vi "RotateX.vi"(8 "error in (no error)":errorcluster, 9 "radians":dbl, 10 "Modelview in":dbl[][](array[numeric])=[[1.0, 0.0, 0.0, 0.0], [0.0, 1.0, 0.0, 0.0], [0.0, 0.0, 1.0, 0.0], [0.0, 0.0, 0.0, 1.0]], 11 "3D Scene in":refnum<class "3D Scene.lvclass">) -> (0 "error out":errorcluster, 2 "Modelview out":dbl[][](array[numeric]), 3 "3D Scene out":refnum<class "3D Scene.lvclass">)   [LabVIEW 2015, in "3D Scene.lvclass"]
uses:
  3D Scene.lvclass
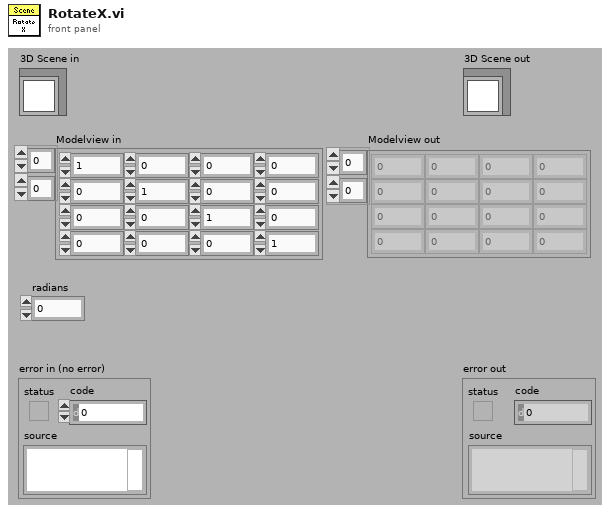
[diagram p1: front panel]
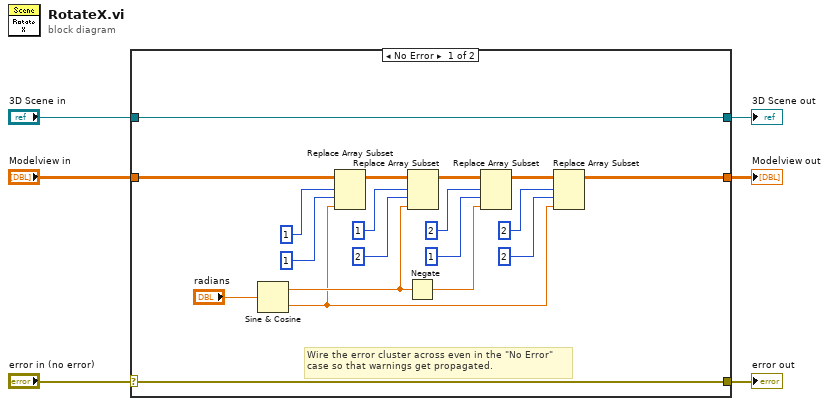
[diagram p0: block diagram]
diagram:
  n1 = case shown="No Error" "error in (no error)" {
    selector: "error in (no error)" -> [w24 w27]
    tunnel: [w24 w27] -> w5
    tunnel: [w25 w26] -> w3
    tunnel: "3D Scene in" -> [w25 w26]
    tunnel: [w8 _] -> w2
    tunnel: "Modelview in" -> [w7 _]
    frame No Error {
      # "Wire the error cluster across even in the \"No Error\"\ncase so that warnings get propagated."
      n2 = Sine & Cosine(0:"radians") -> (1:w12:dbl, 2:w10:dbl)
      n3 = Replace Array Subset(array=w7, new element=w10, index (row)=1, index (col)=1 ("disabled index (col)")) -> (w23:dbl[][])
      n4 = Negate(x=w12) -> (-x=w11:dbl)
      n5 = Replace Array Subset(array=w23, new element=w12, index (row)=1 ("disabled index (row)"), index (col)=2 ("disabled index (col)")) -> (w22:dbl[][])
      n6 = Replace Array Subset(array=w22, new element=w11, index (row)=2, index (col)=1 ("disabled index (col)")) -> (w21:dbl[][])
      n7 = Replace Array Subset(array=w21, new element=w10, index (row)=2, index (col)=2 ("disabled index (col)")) -> (w8:dbl[][])
    }
    frame Error {
    }
  }
  "error out" <- w5
  "3D Scene out" <- w3
  "Modelview out" <- w2
